vi "makedir.vi"(7 "time_stamp":bool, 11 "Path":string) -> (3 "concatenated string 2":string)   [LabVIEW 2012]
panel:
  out "concatenated string":string
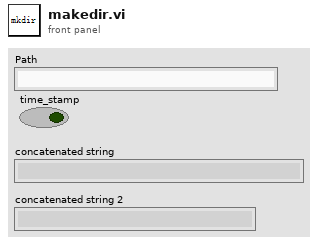
[diagram p1: front panel]
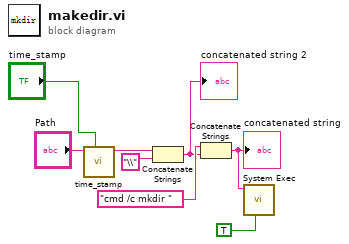
[diagram p0: block diagram]
diagram:
  n1 = call "time_stamp.vi"("time_stamp"="time_stamp", "String in"="Path") -> ("String out"=w7:string)  [unwired: 9 in]
  n2 = Concatenate Strings(w7, "\\" ("字符串")) -> (w1:string)
  "concatenated string 2" <- w1
  n3 = Concatenate Strings("cmd /c mkdir " ("command line"), w1) -> (w3:string)
  "concatenated string" <- w3
  n4 = call <vilib>:"System Exec.vi"("run minimized? (F)"=TRUE, "command line"=w3) -> ()  [unwired: 6 in, 4 out]
